vi "projektlv.vi"() -> ()   [LabVIEW 2023]
doc: "Use this template to build a standard state machine design pattern. Each state executes code and determines which state to transition to. Contrast this design pattern with the User Interface Event Handler pattern, in which code executes in response to user actions. Contrast this design pattern also with the Queued Message Handler pattern, in which each message handling code can queue zero or more new messages.\nNote: This template does not contain the most recent programming guidelines recommended by National Instruments. For a complete, project-based implementation of the Standard State Machine pattern, use the Create Project dialog box instead of this template."
uses:
  projektlv.ctl
  <vilib>/Instr/_visa.llb/VISA Configure Serial Port (Instr).vi
panel:
  in  "Alarm [TEMPERATURA]":dbl(slide) step=10.0 scale=0.0..50.0
  in  "Alarm [WILGOTNOSC]":dbl(slide) step=10.0 scale=0.0..100.0
  in  "stop":bool
  in  "VISA resource name":refnum<visa-resource-name>
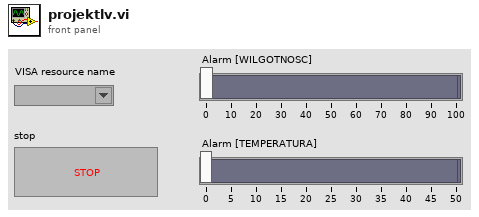
[diagram p1: front panel]
types:
  T1 = typedef "projektlv.ctl" = enum16{"Initialize", "Write", "Send humidity slider", "Send temperature slider", "Stop"}
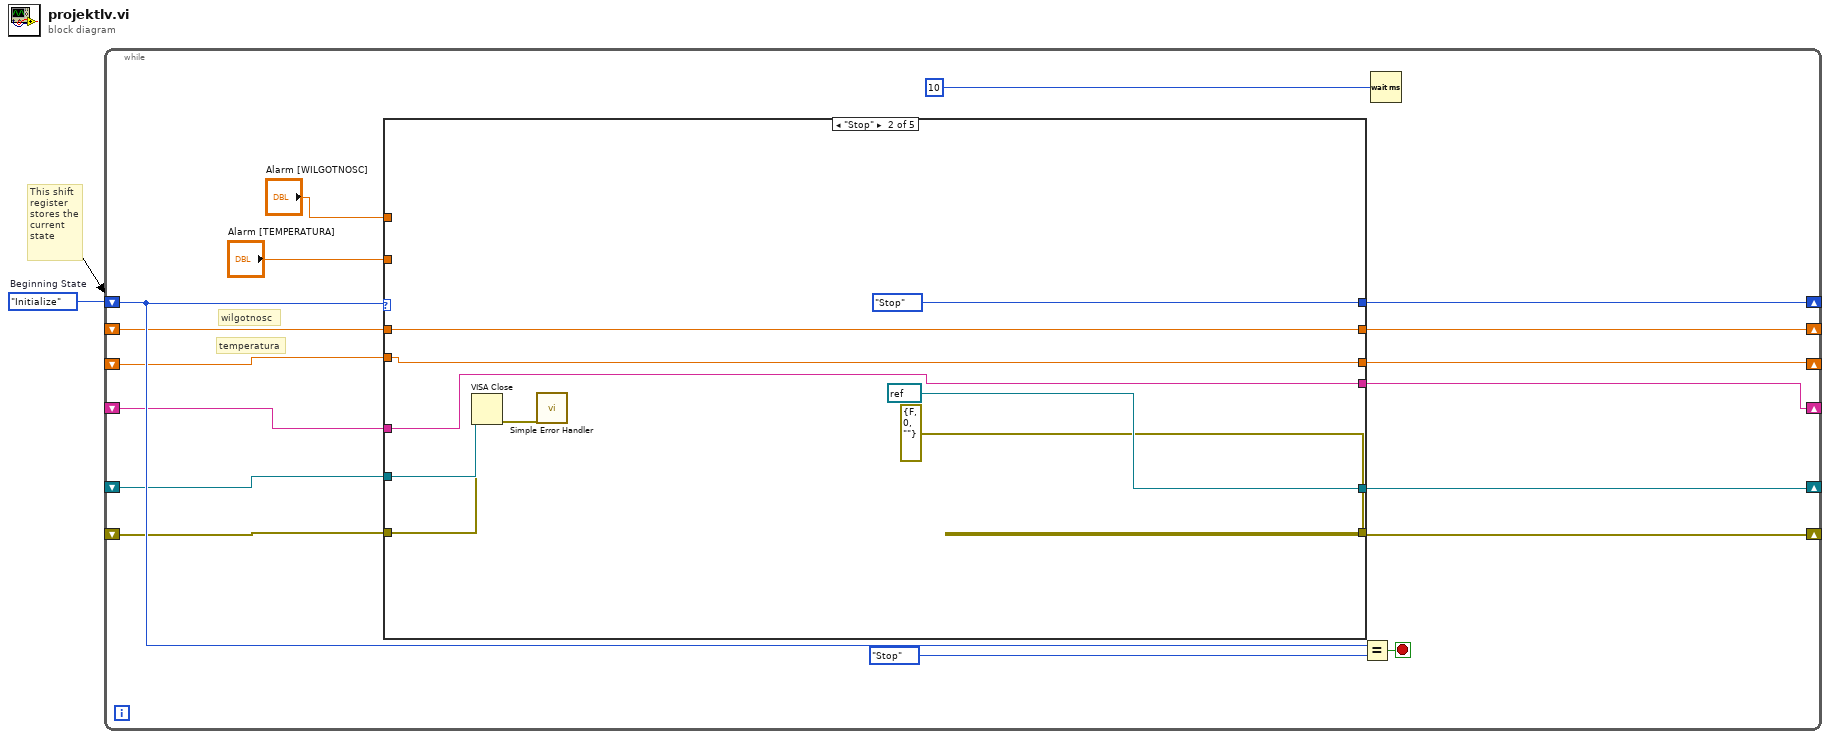
[diagram p0: block diagram]
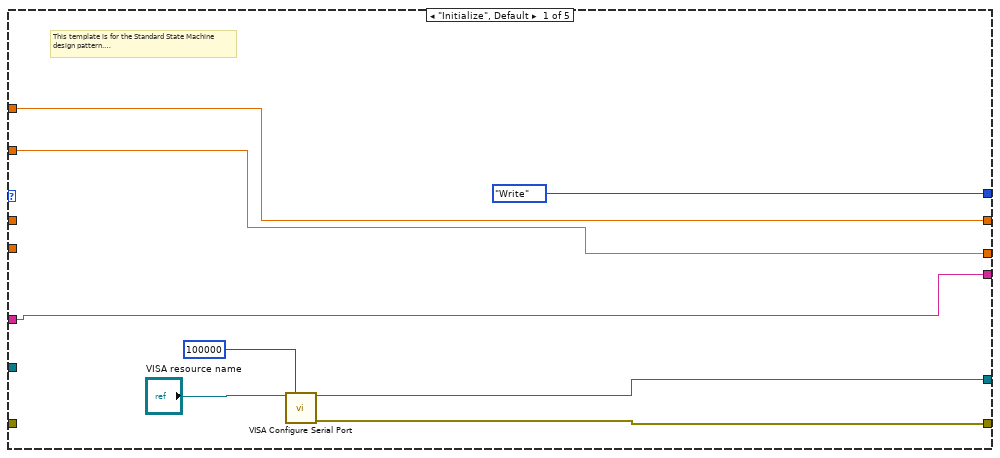
[diagram p2: hidden frame]
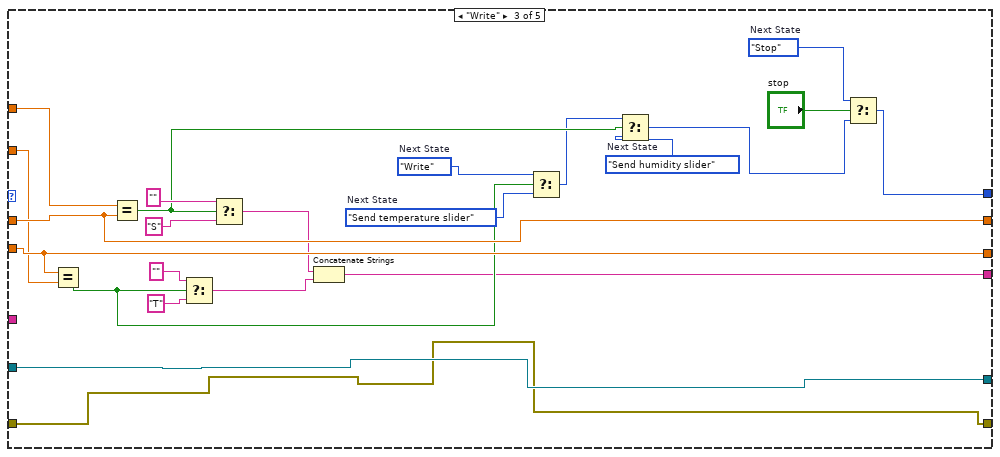
[diagram p3: hidden frame]
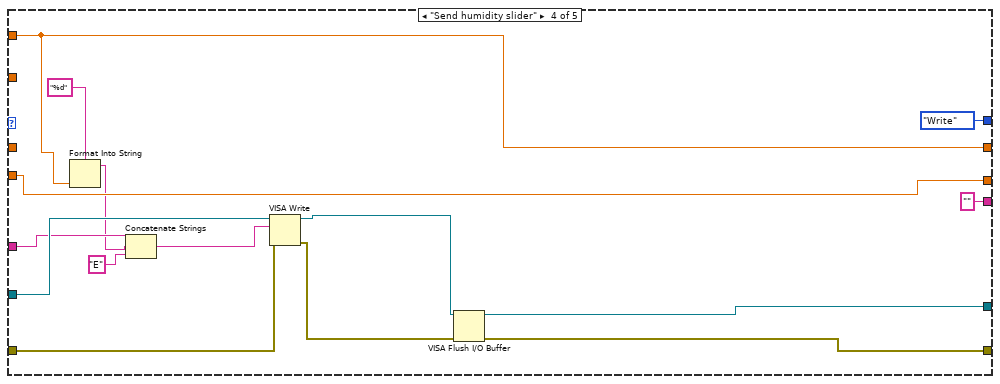
[diagram p4: hidden frame]
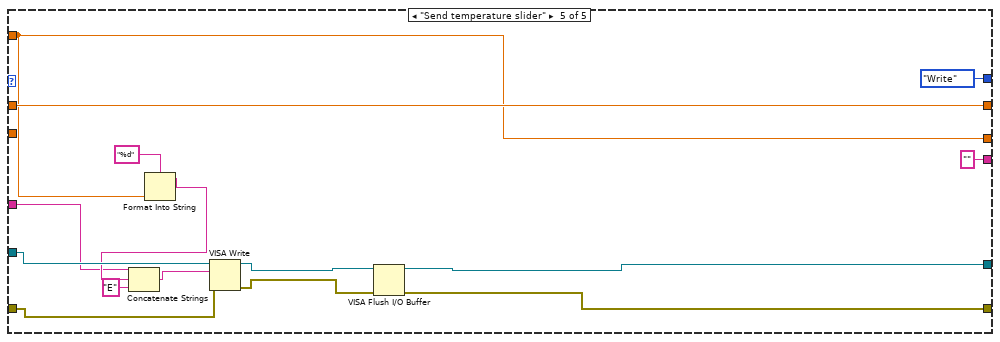
[diagram p5: hidden frame]
diagram:
  w1 = projektlv."Initialize"  # Beginning State
  # "This shift\nregister\nstores the\ncurrent\nstate"
  n1 = while {
    shift-right: [w15] -> _
    shift-left: w1 -> [w16]
    shift-right: [w13] -> _
    shift-left: _ -> [w11]
    shift-right: [w12] -> _
    shift-left: _ -> [w10]
    shift-right: [w8] -> _
    shift-left: _ -> [w7]
    shift-right: [w4] -> _
    shift-left: _ -> [w5]
    shift-right: [w3] -> _
    shift-left: _ -> [w2]
    stop <- w18 stop-if-true
    # "wilgotnosc"
    # "temperatura"
    n2 = case shown="\"Stop\"" w16 {
      tunnel: [projektlv."Write" ("Next State") projektlv."Stop" ("Next State") w56 projektlv."Write" ("Next State") projektlv."Write" ("Next State")] -> w15
      tunnel: [w25 refnum<visa-resource-name> refnum ("VISA resource name out") w37 w67 w82] -> w13
      tunnel: [w24 errorcluster {"status"=FALSE, "code"=0, "source"=""} ("error out") w36 w66 w81] -> w12
      tunnel: w11 -> [_ w34 w37 w73 w86]
      tunnel: w10 -> [_ w33 w36 w72 w85]
      tunnel: "Alarm [WILGOTNOSC]" -> [w21 _ w55 w68 _]
      tunnel: [w21 w29 w50 w68 w88] -> w8
      tunnel: w7 -> [_ w29 w50 _ w88]
      tunnel: "Alarm [TEMPERATURA]" -> [w20 _ w48 _ w83]
      tunnel: w5 -> [_ w28 w49 w69 _]
      tunnel: [w20 w28 w49 w69 w83] -> w4
      tunnel: [w19 w27 w38 "" ""] -> w3
      tunnel: w2 -> [w19 w27 _ w62 w76]
      frame "Initialize", Default {
        # "This template is for the Standard State Machine design pattern.\n\nEach frame of this case structure executes code for its state and\ncomputes what state to transition to next.\n\nStates are represented as values of an enumeration. These enumerations are instances\nof a type definition so that states can be quickly added. To edit the \ntype definition, right click on an enumeration and select Open Type Def."
        n3 = call-poly "VISA Configure Serial Port"("VISA resource name"="VISA resource name", "timeout (10sec)"=u32 100000) -> ("VISA resource name out"=w25:refnum<visa-resource-name>, "error out"=w24:errorcluster)  [unwired: 12 in]
      }
      frame "Stop" {
        n4 = VISA Close(VISA resource name=w34, error in (no error)=w33) -> (error out=w32:errorcluster)
        n5 = call <vilib>:"Simple Error Handler.vi"("error in (no error)"=w32) -> ()  [unwired: 4 in, 5 out]
      }
      frame "Write" {
        w42 = projektlv."Send temperature slider"  # Next State
        w43 = projektlv."Write"  # Next State
        w51 = projektlv."Send humidity slider"  # Next State
        w57 = projektlv."Stop"  # Next State
        n6 = Equal?(x=w49, y=w48) -> (x = y?=w44:bool)
        n7 = Equal?(x=w55, y=w50) -> (x = y?=w47:bool)
        n8 = Select(t="" ("write buffer"), s=w44, f="T" ("write buffer")) -> (s? t:f=w39:string)
        n9 = Select(t="" ("write buffer"), s=w47, f="S" ("write buffer")) -> (s? t:f=w40:string)
        n10 = Concatenate Strings(w40, w39) -> (w38:string)
        n11 = Select(t=w43, s=w44, f=w42) -> (s? t:f=w41:T1)
        n12 = Select(t=w41, s=w47, f=w51) -> (s? t:f=w52:T1)
        n13 = Select(t=w57, s="stop", f=w52) -> (s? t:f=w56:T1)
      }
      frame "Send humidity slider" {
        n14 = Format Into String(format string="%d", w68) -> (resulting string=w61:string)  [unwired: 2 in, 1 out]
        n15 = Concatenate Strings(w62, w61, "E" ("string")) -> (w63:string)
        n16 = VISA Write(VISA resource name=w73, write buffer=w63, error in (no error)=w72) -> (VISA resource name out=w65:refnum<visa-resource-name>, error out=w64:errorcluster)  [unwired: 1 out]
        n17 = VISA Flush I/O Buffer(VISA resource name=w65, error in (no error)=w64) -> (VISA resource name out=w67:refnum<visa-resource-name>, error out=w66:errorcluster)  [unwired: 1 in]
      }
      frame "Send temperature slider" {
        n18 = Format Into String(format string="%d", w83) -> (resulting string=w77:string)  [unwired: 2 in, 1 out]
        n19 = Concatenate Strings(w76, w77, "E" ("string")) -> (w78:string)
        n20 = VISA Write(VISA resource name=w86, write buffer=w78, error in (no error)=w85) -> (VISA resource name out=w80:refnum<visa-resource-name>, error out=w79:errorcluster)  [unwired: 1 out]
        n21 = VISA Flush I/O Buffer(VISA resource name=w80, error in (no error)=w79) -> (VISA resource name out=w82:refnum<visa-resource-name>, error out=w81:errorcluster)  [unwired: 1 in]
      }
    }
    n22 = Equal?(x=w16, y=projektlv."Stop" ("States")) -> (x = y?=w18:bool)
    n23 = Wait (ms)(milliseconds to wait=u32 10) -> ()  [unwired: 1 out]
  }
